vi "Option Parser.vi"(0 "Tektronix PA1000 in":refnum<class "Tektronix PA1000.lvclass">, 1 "ID":string, 2 "THD?":bool, 3 "Number of Cards":dbl, 4 "ID cluster.Model":string, 5 "error in (no error)":errorcluster, 7 "Option":string) -> (14 "Tektronix PA1000 out":refnum<class "Tektronix PA1000.lvclass">, 19 "error out":errorcluster)   [LabVIEW 2013, in "Universal Power Meter.lvlib" / "Tektronix PA1000.lvlib" / "Tektronix PA1000.lvclass"]
uses:
  Tektronix PA1000.lvclass
  Universal Power Meter class/Universal Power Meter.lvclass
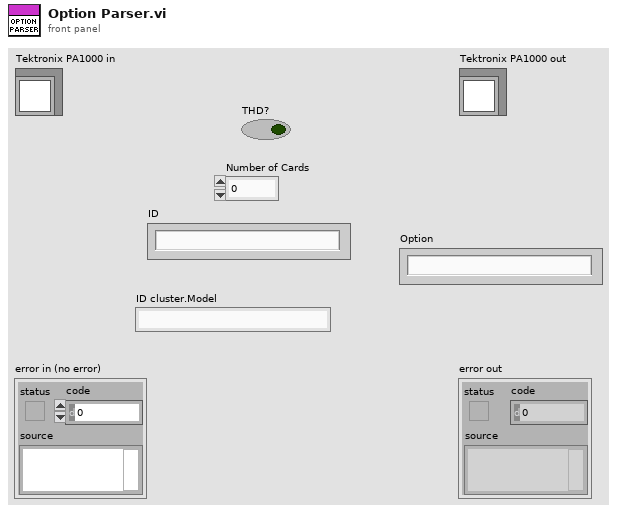
[diagram p1: front panel]
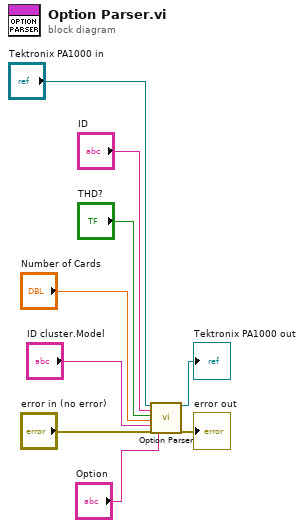
[diagram p0: block diagram]
diagram:
  n1 = call-parent "Option Parser.vi"("Universal Power Meter in"="Tektronix PA1000 in", "ID"="ID", "THD?"="THD?", "Number of Cards"="Number of Cards", "ID cluster.Model"="ID cluster.Model", "error in (no error)"="error in (no error)", "Option"="Option") -> ("Universal Power Meter out"=→"Tektronix PA1000 out":refnum<class "Tektronix PA1000.lvclass">, "error out"=→"error out":errorcluster)  [unwired: 11 in]
